vi "dambing cap.vi"() -> ()   [LabVIEW 2012]
uses:
  <vilib>/Instr/_visa.llb/VISA Configure Serial Port (Instr).vi
panel:
  out "concatenated string 2":string
  out "damping ratio 2":dbl
  out "Cursor.Cursor Position:Cursor X1":dbl
  out "Cursor.Cursor Position:Cursor X2":dbl
  out "Waveform Graph":i32[](graph)
  out "damping ration":dbl
  out "Waveform Chart":i32(graph)
  out "concatenated string":string
  in  "stop":bool
  in  "VISA resource name":refnum<visa-resource-name>
  # "logarithmic decrement"
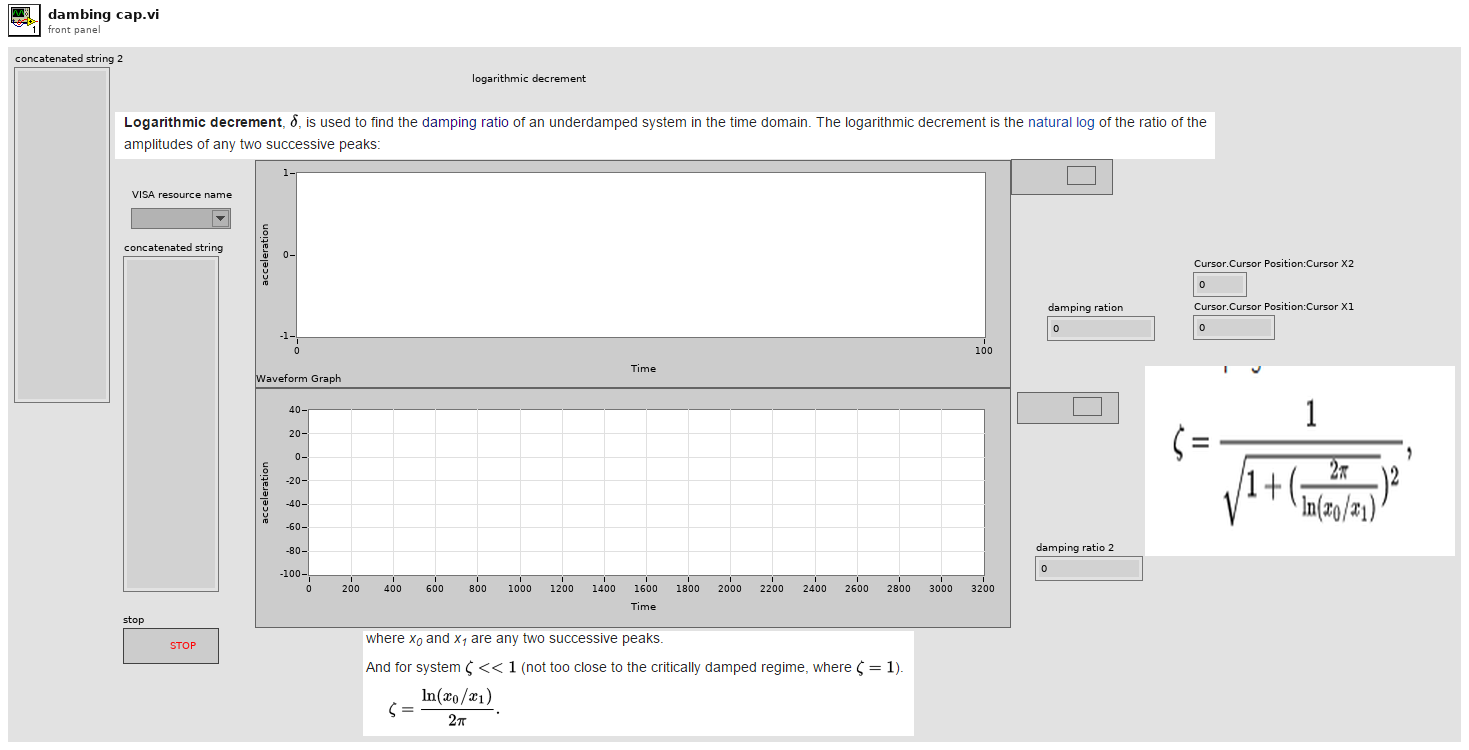
[diagram p1: front panel]
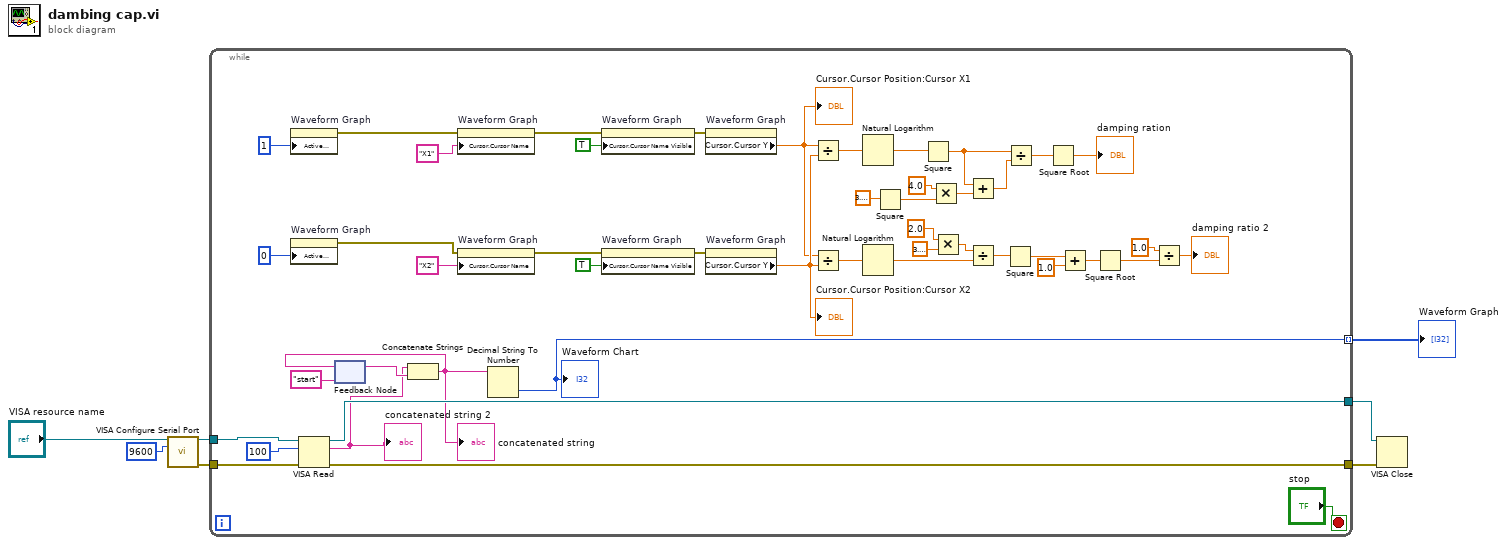
[diagram p0: block diagram]
diagram:
  n1 = call-poly "VISA Configure Serial Port"("VISA resource name"="VISA resource name", "baud rate (9600)"=u32 9600) -> ("VISA resource name out"=w6:refnum<visa-resource-name>, "error out"=w4:errorcluster)  [unwired: 12 in]
  n2 = while {
    tunnel: w6 -> [w48]
    tunnel: [w54] -> w5
    tunnel: w4 -> [w49]
    tunnel: [w53] -> w3
    tunnel: [w35] -> w1 mode=indexing
    stop <- "stop" stop-if-true
    n3 = property on="Waveform Graph" class="WFGraph (strict)"("Active Cursor"=u32 1) -> (error out=w30:errorcluster)  [unwired: 2 in, 1 out]
    n4 = property on="Waveform Graph" class="WFGraph (strict)"("Active Cursor"=u32 0) -> (error out=w27:errorcluster)  [unwired: 2 in, 1 out]
    n5 = VISA Read(VISA resource name=w48, byte count=u32 100, error in (no error)=w49) -> (VISA resource name out=w54:refnum<visa-resource-name>, read buffer=w8:string, error out=w53:errorcluster)  [unwired: 1 out]
    "concatenated string 2" <- w8
    n6 = feedback #1("start") -> (w51:string)
    n7 = Concatenate Strings(w8, w51) -> (w36:string)
    "concatenated string" <- w36
    n8 = feedback-in #1(w36) -> ()
    n9 = property on="Waveform Graph" class="WFGraph (strict)"(error in=w30, "Cursor.Cursor Name"="X1") -> (error out=w32:errorcluster)  [unwired: 1 in, 1 out]
    n10 = property on="Waveform Graph" class="WFGraph (strict)"(error in=w27, "Cursor.Cursor Name"="X2") -> (error out=w25:errorcluster)  [unwired: 1 in, 1 out]
    n11 = Decimal String To Number(string=w36) -> (number=w35:i32)  [unwired: 2 in, 1 out]
    "Waveform Chart" <- w35
    n12 = property on="Waveform Graph" class="WFGraph (strict)"(error in=w32, "Cursor.Cursor Name Visible"=TRUE) -> (error out=w29:errorcluster)  [unwired: 1 in, 1 out]
    n13 = property on="Waveform Graph" class="WFGraph (strict)"(error in=w25, "Cursor.Cursor Name Visible"=TRUE) -> (error out=w28:errorcluster)  [unwired: 1 in, 1 out]
    n14 = property on="Waveform Graph" class="WFGraph (strict)"(error in=w29) -> ("Cursor.Cursor Y"=w9:dbl)  [unwired: 1 in, 2 out]
    "Cursor.Cursor Position:Cursor X1" <- w9
    n15 = property on="Waveform Graph" class="WFGraph (strict)"(error in=w28) -> ("Cursor.Cursor Y"=w10:dbl)  [unwired: 1 in, 2 out]
    "Cursor.Cursor Position:Cursor X2" <- w10
    n16 = Divide(x=w9, y=w10) -> (x/y=w46:dbl)
    n17 = Divide(x=w9, y=w10) -> (x/y=w22:dbl)
    n18 = Natural Logarithm(1:w46) -> (0:w45:dbl)
    n19 = Natural Logarithm(1:w22) -> (0:w18:dbl)
    n20 = Square(x=3.141592653589793) -> (x^2=w42:dbl)
    n21 = Square(x=w45) -> (x^2=w39:dbl)
    n22 = Multiply(x=4.0, y=w42) -> (x*y=w41:dbl)
    n23 = Multiply(x=2.0, y=3.141592653589793) -> (x*y=w19:dbl)
    n24 = Add(x=w39, y=w41) -> (x+y=w40:dbl)
    n25 = Divide(x=w19, y=w18) -> (x/y=w17:dbl)
    n26 = Square(x=w17) -> (x^2=w16:dbl)
    n27 = Divide(x=w39, y=w40) -> (x/y=w38:dbl)
    n28 = Square Root(x=w38) -> (sqrt(x)=→"damping ration":dbl)
    n29 = Add(x=w16, y=1.0) -> (x+y=w14:dbl)
    n30 = Square Root(x=w14) -> (sqrt(x)=w13:dbl)
    n31 = Divide(x=1.0, y=w13) -> (x/y=→"damping ratio 2":dbl)
  }
  "Waveform Graph" <- w1
  n32 = VISA Close(VISA resource name=w5, error in (no error)=w3) -> ()  [unwired: 1 out]
